vi "Get settings chain.vi"(8 "error in (no error)":errorcluster, 11 "LineCCDBase in":refnum<class "LineCCD.lvclass">) -> (0 "error out":errorcluster, 1 "class name":string[](array[string]), 2 "settings":variant[](array[variant]), 3 "LineCCDBase out":refnum<class "LineCCD.lvclass">)   [LabVIEW 2012, in "LineCCD.lvclass"]
doc: "Returns an array of variants containing the settings clusters of each class in the inheritance chain (lowest child class first), together with an array of all class names in the inheritance chain.\n\nFor classes without settings cluster, the settings chain contains empty variants."
uses:
  LineCCD.lvclass
  <vilib>/Distrio/Murmex/Murmex/Murmex.lvclass
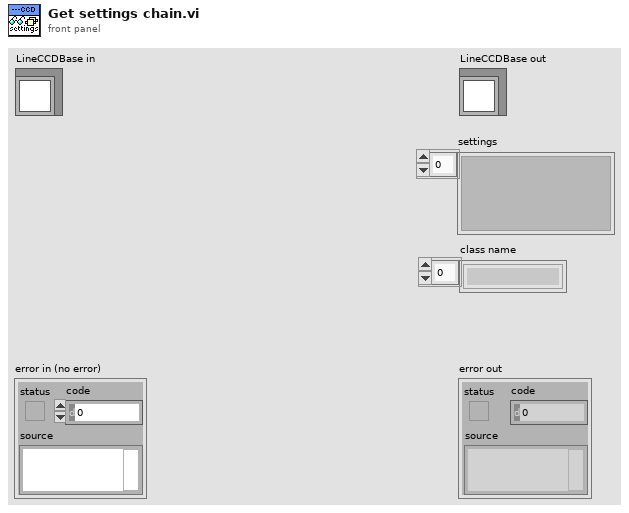
[diagram p1: front panel]
types:
  T1 = typedef "LineCCD.lvclass/settings.ctl" = cluster{"Integration time":dbl[unit], "Scans per Acquisition":u32, "Trig out before integration":dbl[unit], "Enable trig out after config":bool, "Hardware dark correction":bool, "calculate average":bool, "Imaging mode":T2, "file name":string}
  T2 = typedef "Thorcam.lvclass/imaging mode.ctl" = enum16{"free run mode", "single frame"}
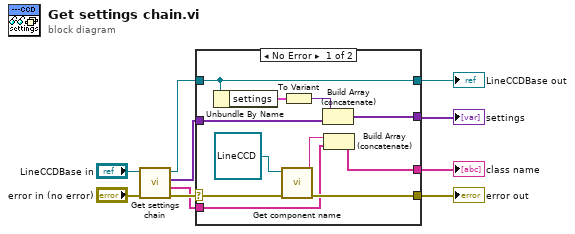
[diagram p0: block diagram]
diagram:
  n1 = call-parent "Get settings chain.vi"("error in (no error)"="error in (no error)", "MurmexBase in"="LineCCDBase in") -> ("error out"=w8:errorcluster, "class name"=w2:string[], "settings"=w3:variant[], "MurmexBase out"=w6:refnum<class "LineCCD.lvclass">)  [unwired: 6 in]
  n2 = case shown="No Error" w8 {
    selector: w8 -> [w19 w23]
    tunnel: [w18 w23] -> w7
    tunnel: w6 -> [w16 w25]
    tunnel: [w16 w25] -> w5
    tunnel: [w15 w24] -> w4
    tunnel: w3 -> [w13 w24]
    tunnel: w2 -> [w12 w22]
    tunnel: [w11 w22] -> w1
    frame No Error {
      n3 = Unbundle By Name(w16) -> ("settings"=w14:T1)
      n4 = call <vilib>:"Get component name.vi"("error in (no error)"=w19, "Murmex in"=refnum<class "LineCCD.lvclass"> refnum ("LineCCD.lvclass")) -> ("error out"=w18:errorcluster, "component name"=w20:string)  [unwired: 7 in, 1 out]
      n5 = To Variant(anything=w14) -> (Variant=w21:variant)
      n6 = Build Array (concatenate)(w21, w13) -> (w15:variant[])
      n7 = Build Array (concatenate)(w20, w12) -> (w11:string[])
    }
    frame Error {
    }
  }
  "error out" <- w7
  "LineCCDBase out" <- w5
  "settings" <- w4
  "class name" <- w1
